vi "Set Channel Wavelength.vi"(1 "Wait until set":bool, 2 "Wavelength (nm)":dbl=750.0, 3 "Channel":i32=1) -> ()   [LabVIEW 2020]
uses:
  Laser Parameters.vi
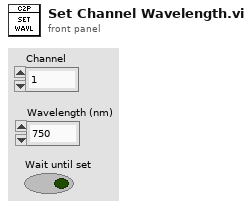
[diagram p1: front panel]
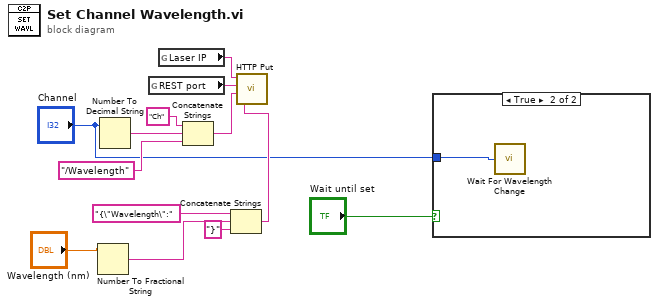
[diagram p0: block diagram]
diagram:
  n1 = Number To Fractional String(number="Wavelength (nm)") -> (F-format string=w6:string)  [unwired: 3 in]
  n2 = Number To Decimal String(number="Channel") -> (decimal integer string=w8:string)  [unwired: 1 in]
  n3 = global read "Laser Parameters.vi" "REST port"() -> (w12:string)
  n4 = global read "Laser Parameters.vi" "Laser IP"() -> (w13:string)
  n5 = Concatenate Strings("Ch" ("Endpoint"), w8, "/Wavelength" ("Endpoint")) -> (w10:string)
  n6 = Concatenate Strings("{\"Wavelength\":" ("string"), w6, "}" ("string")) -> (w3:string)
  n7 = call "HTTP Put.vi"("Buffer"=w3, "Endpoint"=w10, "Port"=w12, "IP Address"=w13) -> ()  [unwired: 2 out]
  n8 = case shown="True" "Wait until set" {
    tunnel: "Channel" -> [_ w14]
    frame False {
    }
    frame True {
      n9 = call "Wait For Wavelength Change.vi"("Channel"=w14) -> ()  [unwired: 1 in]
    }
  }
